vi "Mark Error.vi"(8 "error":errorcluster) -> (0 "marked error":errorcluster, 3 "first time?":bool)   [LabVIEW 2024, in "Logging.lvlib"]
uses:
  Logging.lvlib
panel:
  # "Connector Pane"
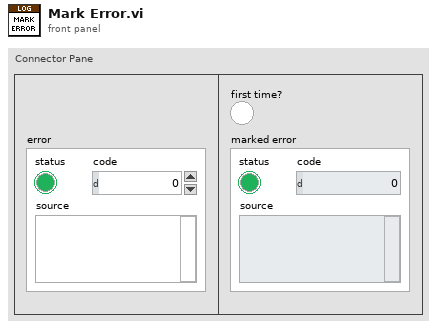
[diagram p1: front panel]
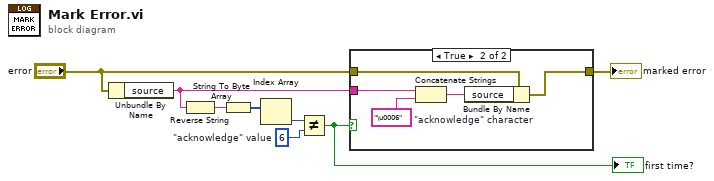
[diagram p0: block diagram]
diagram:
  w4 = u8 6  # "acknowledge" value
  n1 = Unbundle By Name("error") -> ("source"=w3:string)
  n2 = Reverse String(1:w3) -> (0:w2:string)
  n3 = String To Byte Array(string=w2) -> (unsigned byte array=w6:u8[])
  n4 = Index Array(array=w6) -> (element=w5:u8)  [unwired: 1 in]
  n5 = Not Equal?(x=w5, y=w4) -> (x != y?=w1:bool)
  "first time?" <- w1
  n6 = case shown="True" w1 {
    tunnel: "error" -> [w9 w12]
    tunnel: [w9 w11] -> w7
    tunnel: w3 -> [_ w10]
    frame False {
    }
    frame True {
      w14 = "\u0006"  # "acknowledge" character
      n7 = Concatenate Strings(w10, w14) -> (w13:string)
      n8 = Bundle By Name(cluster=w12, "source"=w13) -> (w11:errorcluster)
    }
  }
  "marked error" <- w7
